vi "CREATE OF DB.vi"(8 "errin":errorcluster, 10 "OF":string="00084480_A|1|PCS||091937|", 11 "state":string="1") -> (0 "error out":errorcluster)   [LabVIEW 2020]
doc: "Creer l'OF dans la base"
uses:
  subVI/VarGLO/Global var.vi
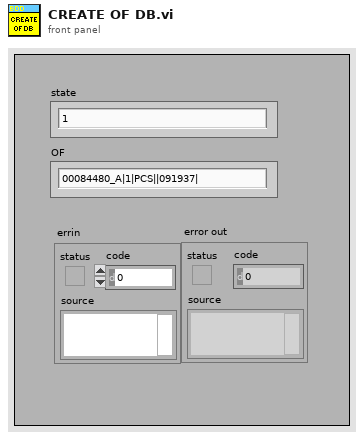
[diagram p1: front panel]
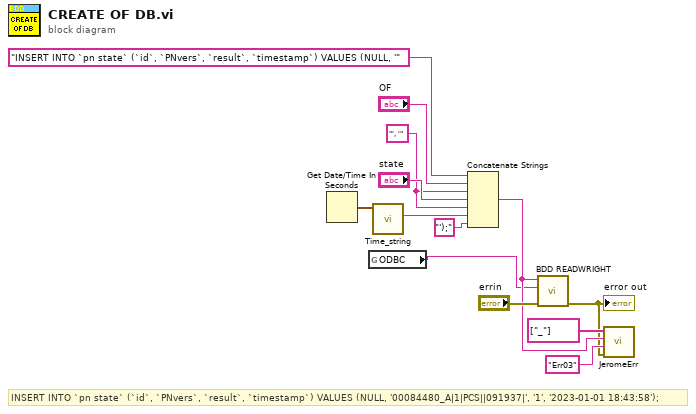
[diagram p0: block diagram]
diagram:
  w8 = "', '" ("chaîne")
  # "INSERT INTO `pn state` (`id`, `PNvers`, `result`, `timestamp`) VALUES (NULL, '00084480_A|1|PCS||091937|', '1', '2023-01-01 18:43:58');"
  n1 = Get Date/Time In Seconds() -> (seconds since 1Jan1904=w10:timestamp)
  n2 = global read "Global var.vi" "ODBC"() -> (w1:string)
  n3 = call <userlib>:"Time_string.vi"("h in"=w10) -> ("heure sql"=w7:string)  [unwired: 9 in, 1 out]
  n4 = Concatenate Strings("INSERT INTO `pn state` (`id`, `PNvers`, `result`, `timestamp`) VALUES (NULL, '" ("SQL query"), "OF", w8, "state", w8, w7, "');" ("chaîne")) -> (w3:string)
  n5 = call <userlib>:"BDD READWRIGHT.vi"("errin"="errin", "DSN name"=w1, "Instruction"=w3) -> ("error out"=w2:errorcluster)  [unwired: 7 in, 1 out]
  "error out" <- w2
  n6 = call "JeromeErr.vi"("Errin"=w2, "CodeERR"="Err03", "RequetteSQL"=w3, "RetourSQL"=string[] ["_"]) -> ()  [unwired: 8 in]
